vi "Calculate Differential.vi"(1 "Idle Offset Voltage":dbl format="%.6g", 2 "Waveform Array In":waveform(dbl)[](array[waveform])) -> (0 "Waveform Out":waveform(dbl))   [LabVIEW 2010]
panel:
  out "Waveforms In":waveform(dbl)[](graph)
  out "Differential (0-1) Waveform Out":waveform(dbl)(graph)
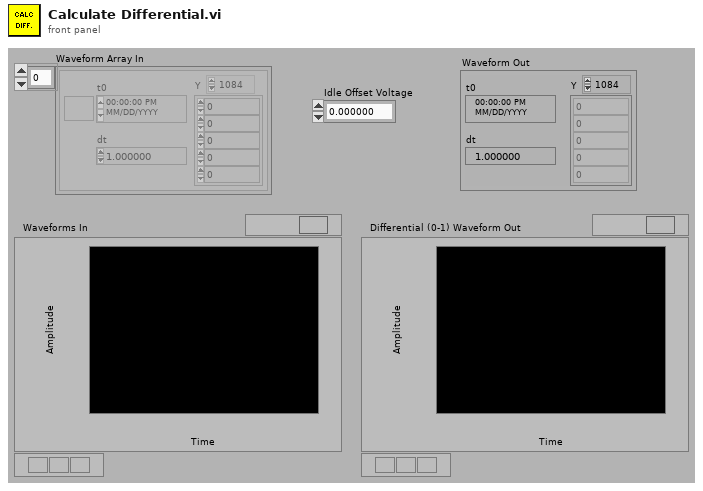
[diagram p1: front panel]
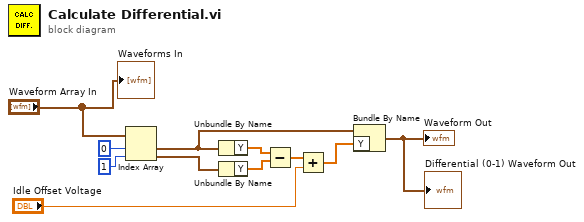
[diagram p0: block diagram]
diagram:
  n1 = Index Array(array="Waveform Array In", index #1=0 ("index"), index #2=1 ("index")) -> (element #1=w3:waveform(dbl), element #2=w9:waveform(dbl))
  n2 = Unbundle By Name(w3) -> ("Y"=w8:dbl[])
  n3 = Unbundle By Name(w9) -> ("Y"=w7:dbl[])
  n4 = Subtract(x=w8, y=w7) -> (x-y=w6:dbl[])
  n5 = Add(x=w6, y="Idle Offset Voltage") -> (x+y=w4:dbl[])
  n6 = Bundle By Name(cluster=w3, "Y"=w4) -> (→"Waveform Out" →"Differential (0-1) Waveform Out":waveform(dbl))
  "Waveforms In" <- "Waveform Array In"
